vi "Part ID.vi"(8 "error in (no error)":errorcluster, 11 "Thermistor1 in":refnum<class "Thermistor1.lvclass">) -> (0 "error out":errorcluster, 1 "Part ID":string, 3 "Thermistor1 out":refnum<class "Thermistor1.lvclass">)   [LabVIEW 2021, in "Thermistor1.lvclass"]
uses:
  Thermistor1.lvclass
  Thermistor1.lvclass/Thermistor1.ctl
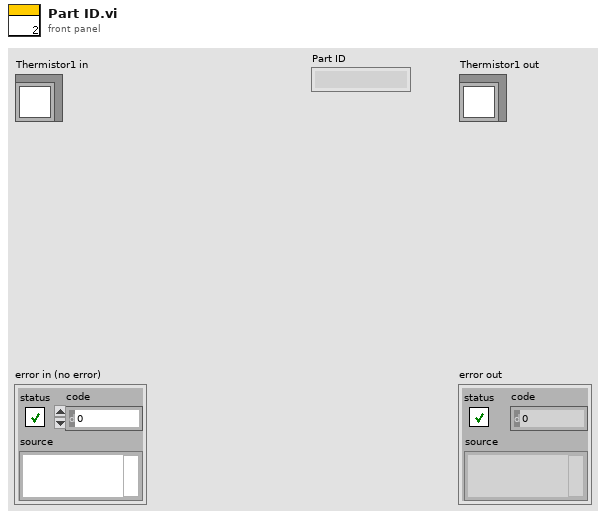
[diagram p1: front panel]
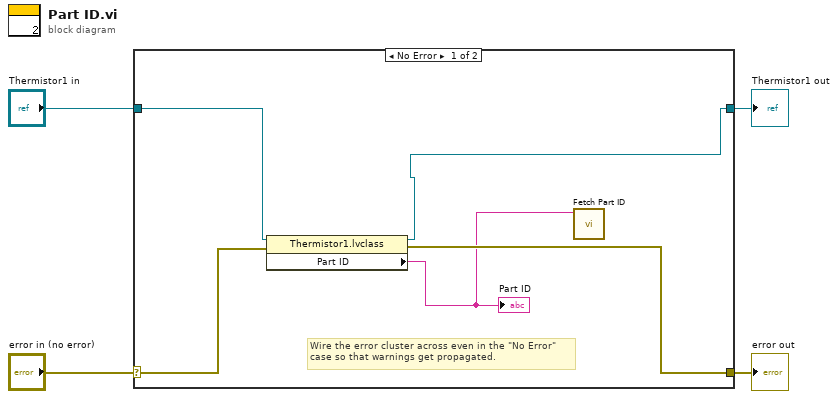
[diagram p0: block diagram]
diagram:
  n1 = case shown="No Error" "error in (no error)" {
    selector: "error in (no error)" -> [w7 w11]
    tunnel: [w6 w11] -> w3
    tunnel: [w8 w10] -> w1
    tunnel: "Thermistor1 in" -> [w9 w10]
    frame No Error {
      # "Wire the error cluster across even in the \"No Error\"\ncase so that warnings get propagated."
      n2 = property class="Thermistor1.lvclass"(reference=w9, error in=w7) -> (reference out=w8:refnum<class "Thermistor1.lvclass">, error out=w6:errorcluster, "Part ID"=w5:string)
      "Part ID" <- w5
      n3 = call "Fetch Part ID.vi"("String"=w5) -> ()  [unwired: 10 in, 1 out]
    }
    frame Error {
    }
  }
  "error out" <- w3
  "Thermistor1 out" <- w1
